vi "Abort Dynamic Generation.vi"(0 "RFSG handle":refnum<k15>, 5 "Timeout (ms)":dbl=1000.0 format="%#_6p", 11 "error in (no error)":errorcluster) -> (4 "RFSG handle out":refnum<k15>, 15 "error out":errorcluster)   [LabVIEW 2018, in "SG.lvlib"]
uses:
  SG.lvlib
  <instrlib>/niRFSG/niRFSG.llb/niRFSG Script Trigger IDs.ctl
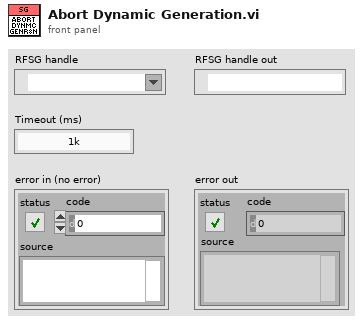
[diagram p1: front panel]
types:
  T1 = typedef "niRFSG Script Trigger IDs.ctl" = string
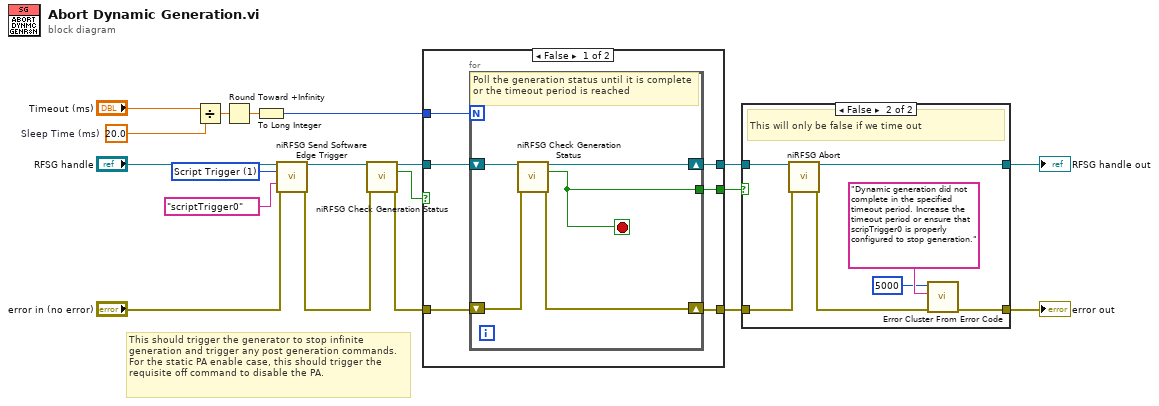
[diagram p0: block diagram]
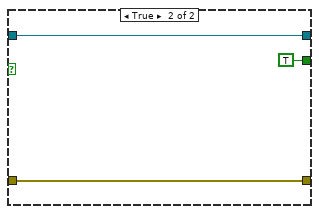
[diagram p3: hidden frame]
diagram:
  w12 = 20.0  # Sleep Time (ms)
  w17 = 1 items=["Start Trigger", "Script Trigger"] ("trigger type")
  # "This should trigger the generator to stop infinite generation and trigger any post generation commands. For the static PA enable case, this should trigger the requisite off command to disable the PA."
  n1 = Divide(x="Timeout (ms)", y=w12) -> (x/y=w13:dbl)
  n2 = Round Toward +Infinity(x=w13) -> (ceil(x): smallest int >= x=w6:dbl)
  n3 = To Long Integer(number=w6) -> (32bit integer=w5:i32)
  n4 = call <instrlib>:"niRFSG Send Software Edge Trigger.vi"("instrument handle"="RFSG handle", "trigger type"=w17, "trigger ID"=T1 "scriptTrigger0", "error in"="error in (no error)") -> ("instrument handle out"=w18:refnum<k15>, "error out"=w11:errorcluster)  [unwired: 10 in]
  n5 = call <instrlib>:"niRFSG Check Generation Status.vi"("instrument handle"=w18, "error in"=w11) -> ("instrument handle out"=w10:refnum<k15>, "done?"=w7:bool, "error out"=w8:errorcluster)  [unwired: 11 in]
  n6 = case shown="False" w7 {
    tunnel: w10 -> [w25 w33]
    tunnel: [w24 w33] -> w9
    tunnel: w8 -> [w23 w32]
    tunnel: [w22 w32] -> w3
    tunnel: w5 -> [w21 _]
    tunnel: [w20 TRUE ("done?")] -> w1
    frame False {
      n7 = for {
        N: w21 -> [_]
        shift-right: [w29] -> w24
        shift-left: w25 -> [w30]
        shift-right: [w27] -> w22
        shift-left: w23 -> [w28]
        tunnel: [w26] -> w20
        stop <- w26 stop-if-true
        # "Poll the generation status until it is complete or the timeout period is reached"
        n8 = call <instrlib>:"niRFSG Check Generation Status.vi"("instrument handle"=w30, "error in"=w28) -> ("instrument handle out"=w29:refnum<k15>, "done?"=w26:bool, "error out"=w27:errorcluster)  [unwired: 11 in]
      }
    }
    frame True {
    }
  }
  n9 = case shown="False" w1 {
    tunnel: w9 -> [w35 w41]
    tunnel: [w35 w40] -> w4
    tunnel: w3 -> [w34 w39]
    tunnel: [w34 w37] -> w2
    frame True {
    }
    frame False {
      # "This will only be false if we time out"
      n10 = call <instrlib>:"niRFSG Abort.vi"("instrument handle"=w41, "error in"=w39) -> ("instrument handle out"=w40:refnum<k15>, "error out"=w38:errorcluster)  [unwired: 12 in]
      n11 = call <vilib>:"Error Cluster From Error Code.vi"("error in (no error)"=w38, "error message (\"\")"="Dynamic generation did not complete in the specified timeout period. Increase the timeout period or ensure that scripTrigger0 is properly configured to stop generation.", "error code (0)"=5000) -> ("error out"=w37:errorcluster)  [unwired: 6 in]
    }
  }
  "RFSG handle out" <- w4
  "error out" <- w2
